vi "Build Low Priority Execute.vi"(6 "Group":i32, 7 "Virtual Memory Unit in":refnum<class "Virtual Memory Unit.lvclass">, 8 "error in (no error)":errorcluster, 10 "Starting Address":u16 format="%04x", 11 "Major Frame in":refnum<class "Major Frame.lvclass">) -> (0 "error out":errorcluster, 2 "Next Available Address":u16 format="%04x", 3 "Major Frame out":refnum<class "Major Frame.lvclass">, 5 "Virtual Memory Unit out":refnum<class "Virtual Memory Unit.lvclass">)   [LabVIEW 2020, in "BCI-1553 API.lvlib" / "Major Frame.lvclass"]
doc: "Creates the execution block for the low priority asynchronous messages.\n\nThis is always an unconditional execute, followed by resetting the group flag, and then returning from the subroutine."
uses:
  Major Frame.lvclass
  Dependencies/Virtual Memory Unit/Virtual Memory Unit.lvclass
  TypeDefs/BC Op Codes - Verbose.ctl
  TypeDefs/BC Condition Codes.ctl
  Major Frame.lvclass/Major Frame.ctl
  BCI-1553 API.lvlib
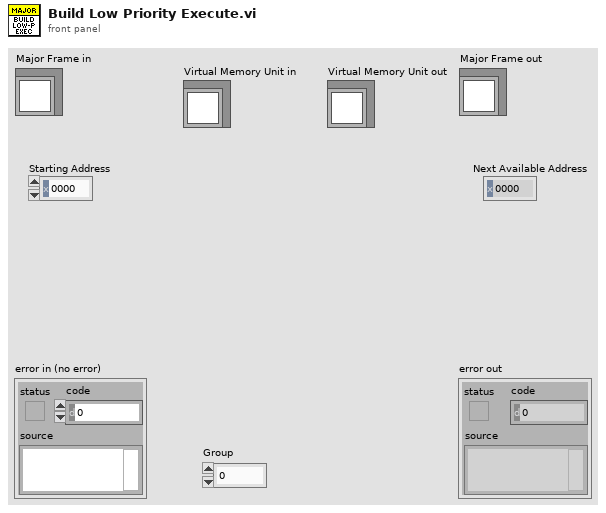
[diagram p1: front panel]
types:
  T1 = typedef "BCI-1553 API.lvlib/BC Condition Codes.ctl" = enum16{"GP0 == 1 || LT", "GP1 == 1 || NE", "GP2 == 1", "GP3 == 1", "GP4 == 1", "GP5 == 1", "GP6 == 1", "GP7 == 1", "NORESP", "FMTERR", "GOODBLOCK", "MSKSTATSET", "BADMSG", "1RETRY", "2RETRY", "ALWAYS"}
  T2 = typedef "BCI-1553 API.lvlib/BC Op Codes - Verbose.ctl" = enum16{"EXECUTE MSG", "EXECUTE MSG GO", "JUMP", "CALL SUBROUTINE", "RETURN", "INTERRUPT REQUEST", "HALT", "DELAY", "WAIT FRAME TIMER = 0", "COMPARE FRAME TIMER", "COMPARE MSG TIMER", "LOAD TIME TAG CTR", "LOAD TIME TAG CTR HI", "LOAD FRAME TIMER", "START FRAME TIMER", "PUSH TIME TAG COUNT", "PUSH TIME TAG COUNT HI", "PUSH TIME TAG COUNT BOTH", "PUSH BLOCK STATUS WORD", "PUSH CURRENT VALUE", "PUSH INDIRECT", "WAIT EXT TRIGGER", "EXECUTE AND FLIP", "EXECUTE, FLIP, GO", "WRITE VALUE TO WMI", "WRITE VALUE TO MEM", "DECREMENT RAM, SKIP", "FLAG"}
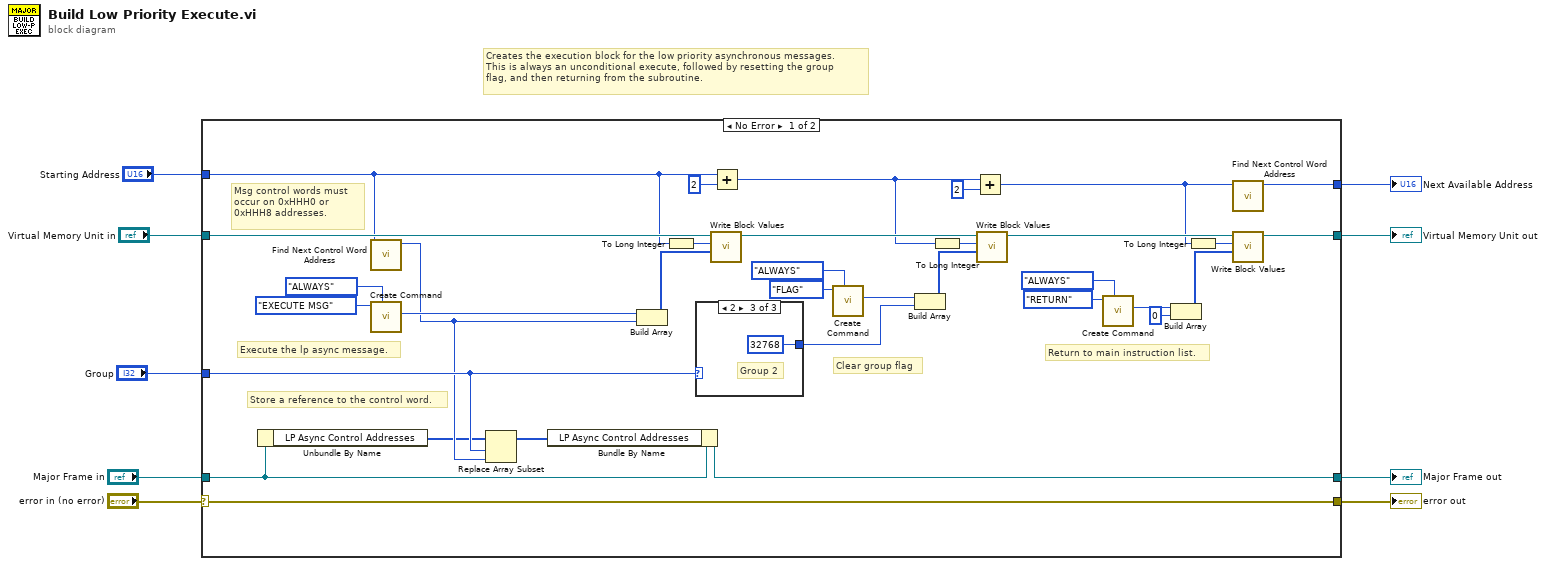
[diagram p0: block diagram]
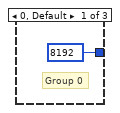
[diagram p2: hidden frame]
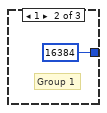
[diagram p3: hidden frame]
diagram:
  # "Creates the execution block for the low priority asynchronous messages.\nThis is always an unconditional execute, followed by resetting the group\nflag, and then returning from the subroutine."
  n1 = case shown="No Error" "error in (no error)" {
    selector: "error in (no error)" -> [w14 w48]
    tunnel: [w14 w48] -> w1
    tunnel: [w15 w47] -> w2
    tunnel: "Major Frame in" -> [w16 w47]
    tunnel: "Virtual Memory Unit in" -> [w41 _]
    tunnel: [w30 _] -> w4
    tunnel: "Starting Address" -> [w17 _]
    tunnel: [w18 _] -> w3
    tunnel: "Group" -> [w13 _]
    frame No Error {
      # "Store a reference to the control word."
      # "Msg control words must\noccur on 0xHHH0 or \n0xHHH8 addresses."
      # "Clear group flag"
      # "Return to main instruction list."
      # "Execute the lp async message."
      n2 = Unbundle By Name(w16) -> ("LP Async Control Addresses"=w11:u16[])
      n3 = call "Find Next Control Word Address.vi"("Starting Address"=w17) -> ("0xHHHX Address"=w12:u16)  [unwired: 10 in]
      n4 = call "Create Command.vi"("Condition"=BC_Condition_Codes."ALWAYS", "Op Code"=BC_Op_Codes_-_Verbose."EXECUTE MSG") -> ("Instruction"=w40:u16)  [unwired: 8 in, 1 out]
      n5 = Replace Array Subset(array=w11, new element=w12, index=w13) -> (w10:u16[])
      n6 = Bundle By Name(cluster=w16, "LP Async Control Addresses"=w10) -> (w15:refnum<class "Major Frame.lvclass">)
      n7 = Build Array(w40, w12) -> (w39:u16[])
      n8 = To Long Integer(number=w17) -> (32bit integer=w38:i32)
      n9 = case shown="2" w13 {
        tunnel: [u16 8192 ("element") u16 16384 ("element") u16 32768 ("element")] -> w20
        frame 0, Default {
          # "Group 0"
        }
        frame 1 {
          # "Group 1"
        }
        frame 2 {
          # "Group 2"
        }
      }
      n10 = call "Write Block Values.vi"("Write Block"=w39, "Start Index"=w38, "Virtual Memory Unit in"=w41) -> ("Virtual Memory Unit out"=w24:refnum<class "Virtual Memory Unit.lvclass">)  [unwired: 7 in, 1 out]
      n11 = Add(x=w17, y=u16 2) -> (x+y=w21:u16)
      n12 = call "Create Command.vi"("Condition"=BC_Condition_Codes."ALWAYS", "Op Code"=BC_Op_Codes_-_Verbose."FLAG") -> ("Instruction"=w27:u16)  [unwired: 8 in, 1 out]
      n13 = Build Array(w27, w20) -> (w28:u16[])
      n14 = To Long Integer(number=w21) -> (32bit integer=w29:i32)
      n15 = Add(x=w21, y=u16 2) -> (x+y=w19:u16)
      n16 = call "Write Block Values.vi"("Write Block"=w28, "Start Index"=w29, "Virtual Memory Unit in"=w24) -> ("Virtual Memory Unit out"=w23:refnum<class "Virtual Memory Unit.lvclass">)  [unwired: 7 in, 1 out]
      n17 = call "Create Command.vi"("Condition"=BC_Condition_Codes."ALWAYS", "Op Code"=BC_Op_Codes_-_Verbose."RETURN") -> ("Instruction"=w32:u16)  [unwired: 8 in, 1 out]
      n18 = Build Array(w32, u16 0 ("element")) -> (w34:u16[])
      n19 = To Long Integer(number=w19) -> (32bit integer=w33:i32)
      n20 = call "Find Next Control Word Address.vi"("Starting Address"=w19) -> ("0xHHHX Address"=w18:u16)  [unwired: 10 in]
      n21 = call "Write Block Values.vi"("Write Block"=w34, "Start Index"=w33, "Virtual Memory Unit in"=w23) -> ("Virtual Memory Unit out"=w30:refnum<class "Virtual Memory Unit.lvclass">)  [unwired: 7 in, 1 out]
    }
    frame Error {
    }
  }
  "error out" <- w1
  "Major Frame out" <- w2
  "Next Available Address" <- w3
  "Virtual Memory Unit out" <- w4
